vi "automated_scan_v1.0.vi"() -> ()   [LabVIEW 2018]
uses:
  Other_Libraries/MoCo Software/VI/global_m.vi
  <vilib>/Utility/file.llb/Write Delimited Spreadsheet (DBL).vi
  <vilib>/Utility/file.llb/Write Delimited Spreadsheet (string).vi
  Other_Libraries/Thorlabs_FW102C/Thorlabs_FW102C.lvlib
panel:
  out "End scan":errorcluster
  out "nloops":i32
  out "FW Position":i32
  out "Filter Wheel":errorcluster
  out "Current Wavelength(nm)":dbl
  out "Take Image":errorcluster
  out "Dark Integrating Time (s)":dbl caption="Elapsed Time (s)"
  out "% complete":dbl
  out "Total Steps":dbl
  in  "Tab Control":T1(tab)
  in  "Photodiode (VISA resource name)[Com3]":refnum<visa-resource-name>="COM3"
  in  "Mono port":refnum<visa-resource-name>="COM2"
  in  "Grating, gr/mm":u16(ring)=2 items=["2400", "1800", "1200", "600", "300", "150"]
  in  "Take Image":bool=TRUE
  in  "Two Cameras":bool=TRUE
  in  "Step Size":dbl=10.0
  in  "Stop Wavelength":dbl=600.0
  in  "Start Wavelength":dbl=500.0
  in  "Scan Directory":string="Peter_ferguson\\Tcal\\scans\\"
  in  "Scan Name":string="test_scan"
  in  "Scan Type":string(combo)="New Scan"
  in  "Photodiode / Camera\n Integration time(s)":dbl=10.0
  in  "Spectrometer Integration time":dbl=0.001
  out "VISA out":refnum<visa-resource-name>
  out "Current Value Bin":dbl format="%.6f"
  out "dup VISA session":refnum<visa-resource-name>
  out "dup VISA session 2":refnum<visa-resource-name>
  out "Mono wav":dbl format="%.3f"
  out "Photodiode 2":errorcluster
  out "Light Integrating Time (s)":dbl caption="Elapsed Time (s)"
  out "Active Wavelength":u32
  out "Serial Number":string
  out "Mono/Photodiode":errorcluster
  out "Step #":i32
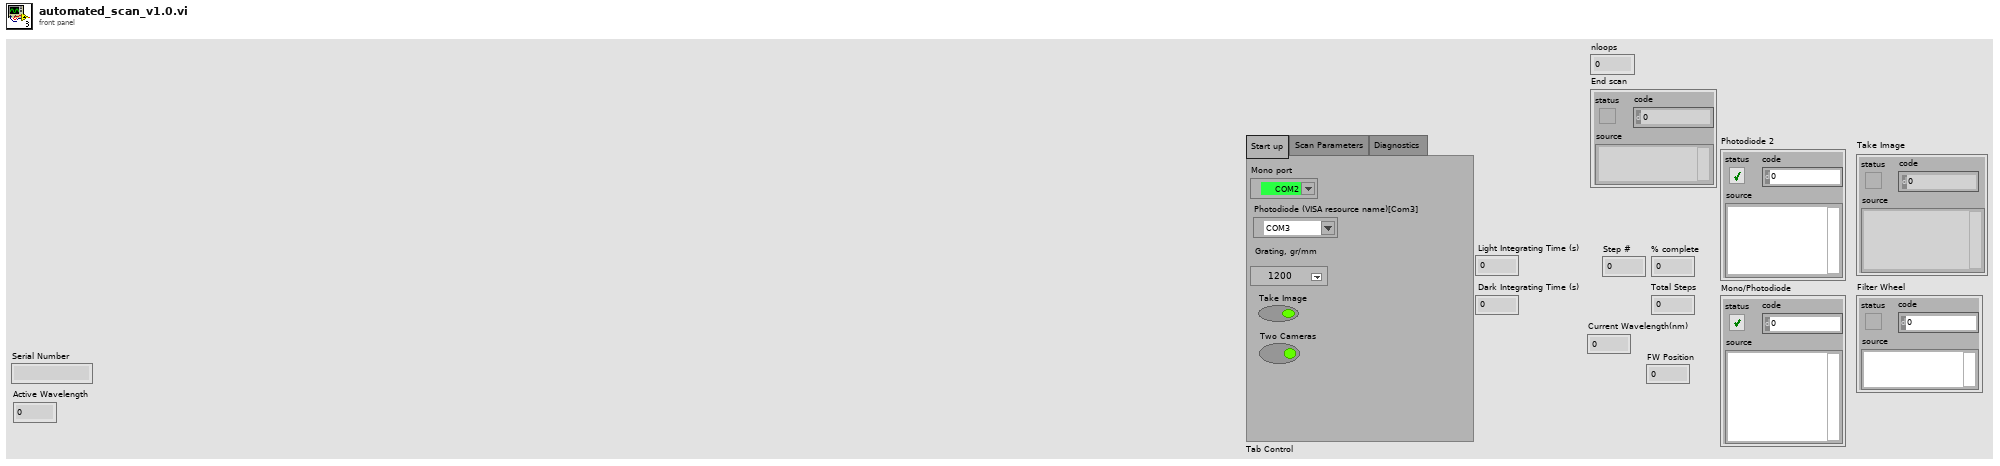
[diagram p1: front panel]
types:
  T1 = enum32{"Start up", "Scan Parameters", "Diagnostics"}
  T2 = cluster{"Head Type":u32, "Head Version":u32, "Serial Number":string, "Calibration Sensitivity":dbl, "Default Wavelength":u32, "Active Sensitivity":dbl, "Active Wavelength":u32, "Scale Min Power (Wattmeter)":u32, "Scale Max Power (Wattmeter)":u32, "Scale Min Energy":u32, "Scale Max Energy":u32, "Current Scale":u32, "Calo Mode":bool, "Anticipation":bool, "External Trig":bool, "Trig Level":dbl, "Zero Offset":dbl, "Multiplier 1":dbl, "Offset 1":dbl, "Multiplier 2":dbl, "Offset 2":dbl, "Max Power (Joulemeter)":dbl, "Max energy (Joulemeter)":dbl, "Currently Logging":bool, "Analog Out Active":bool, "Resolution":dbl, "Currently Calculating Stats":bool, "High-Resolution Display":bool, "Scale Min Wavelenght":u32, "Scale Max Wavelenght":u32, "Upper Bound":dbl, "Lower Bond":dbl, "Reference Value":dbl, "Thresholds Active":bool, "Fail":bool, "Attenuator":bool, "autoScale":bool, "IsdBm":bool}
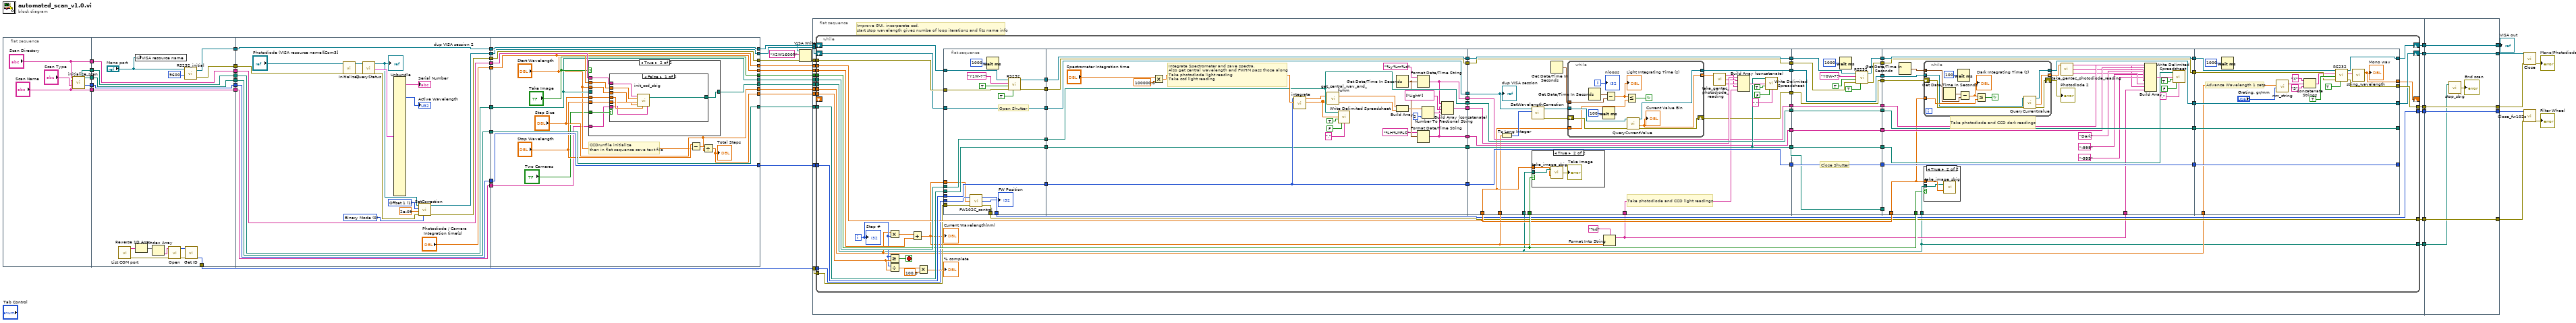
[diagram p0: block diagram]
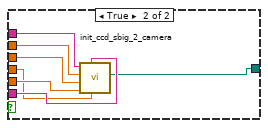
[diagram p5: hidden frame]
diagram:
  n1 = flat-sequence {
    tunnel: [w55] -> w38
    tunnel: [w54] -> w37
    tunnel: [w53] -> w36
    tunnel: ["Scan Directory"] -> w22
    tunnel: ["Scan Name"] -> w7
    tunnel: [w71] -> w35
    tunnel: [w70] -> w34
    tunnel: w38 -> [w69]
    tunnel: [w69] -> w33
    tunnel: w37 -> [w68]
    tunnel: [w68] -> w32
    tunnel: w36 -> [w67]
    tunnel: [w67] -> w31
    tunnel: w22 -> [w66]
    tunnel: [w66] -> w20
    tunnel: [w59] -> w14
    tunnel: [w58] -> w13
    tunnel: [w57] -> w8
    tunnel: w7 -> [w57]
    tunnel: w35 -> [w87]
    tunnel: [w87] -> w30
    tunnel: w34 -> [w83]
    tunnel: w33 -> [w86]
    tunnel: [w86] -> w29
    tunnel: w32 -> [w85]
    tunnel: [w85] -> w28
    tunnel: w31 -> [w84]
    tunnel: [w84] -> w27
    tunnel: [w80] -> w26
    tunnel: ["Photodiode / Camera\n Integration time(s)"] -> w25
    tunnel: [w76] -> w24
    tunnel: [w82] -> w21
    tunnel: w20 -> [w82]
    tunnel: [w74] -> w9
    tunnel: w8 -> [w74]
    tunnel: [w109] -> w40
    tunnel: w30 -> [w109]
    tunnel: [w99] -> w48
    tunnel: w29 -> [w99]
    tunnel: [w108] -> w47
    tunnel: w28 -> [w108]
    tunnel: [w107] -> w46
    tunnel: w27 -> [w107]
    tunnel: [w106] -> w45
    tunnel: w26 -> [w106]
    tunnel: [w103] -> w44
    tunnel: w25 -> [w103]
    tunnel: [w110] -> w39
    tunnel: w24 -> [w105]
    tunnel: [w105] -> w23
    tunnel: w21 -> [w104]
    tunnel: [w101] -> w19
    tunnel: ["Take Image"] -> w18
    tunnel: ["Step Size"] -> w16
    tunnel: ["Start Wavelength"] -> w15
    tunnel: w9 -> [w95]
    frame #0 {
      n2 = call "initialize_scan.vi"("Scan Directory"="Scan Directory", "Scan Name"="Scan Name", "Scan Type"="Scan Type") -> ("Path Spec"=w55:path, "Path Scan"=w53:path, "Wrapper Out"=w54:u64)  [unwired: 8 in, 2 out]
    }
    frame #1 {
      n3 = call "List COM port.vi"() -> ("error out"=w60:errorcluster, "COM Ports"=w63:string[])  [unwired: 10 in]
      n4 = global write "global_m.vi" "VISA resource name"("Mono port") -> ()
      n5 = Reverse 1D Array(array=w63) -> (reversed array=w62:string[])
      n6 = Index Array(array=w62) -> (element=w61:string)  [unwired: 1 in]
      n7 = call "Open.vi"("error in (no error)"=w60, "Serial Port"=w61) -> ("error out"=w64:errorcluster, "FW102C out"=w65:i32)  [unwired: 7 in, 1 out]
      n8 = call "RS232_initial.vi"("baud rate"=u32 9600, "VISA resource name"="Mono port") -> ("error out"=w70:errorcluster, "VISA name out"=w71:refnum<visa-resource-name>)  [unwired: 2 in]
      n9 = call "Get ID.vi"("error in (no error)"=w64, "FW102C in"=w65) -> ("error out"=w58:errorcluster, "FW102C out"=w59:i32)  [unwired: 7 in, 1 out]
    }
    frame #2 {
      w75 = u16 0 items=["Binary Mode", "Text Mode"] ("Transfer Type (binary)")
      w79 = u16 1 items=["Multiplier1", "Offset 1", "Multiplier 2", "Offset 2"] ("Correction Type")
      n10 = call "Initialize2.vi"("error in (no error)"=w83, "Instr. Descriptor (GPIB::)"="Photodiode (VISA resource name)[Com3]") -> ("error out"=w89:errorcluster, "VISA session"=w93:refnum<visa-resource-name>)  [unwired: 4 in]
      n11 = call "QueryStatus.vi"("error in (no error)"=w89, "VISA session"=w93) -> ("error out"=w77:errorcluster, "Status Data"=w92:T2, "dup VISA session"=w81:refnum<visa-resource-name>)  [unwired: 4 in, 1 out]
      "dup VISA session 2" <- w81
      n12 = Unbundle(w92) -> ("Serial Number"=→"Serial Number":string, "Active Wavelength"=→"Active Wavelength":u32)  [unwired: 36 out]
      n13 = call "SetCorrection.vi"("Transfer Type (binary)"=w75, "error in (no error)"=w77, "Correction  Value"=2e-09, "Correction Type"=w79, "VISA session"=w81) -> ("error out"=w76:errorcluster, "dup VISA session"=w80:refnum<visa-resource-name>)  [unwired: 3 in]
    }
    frame #3 {
      # "CCDrunfile initialize\nthen in flat sequence save text file"
      n14 = case shown="True" "Take Image" {
        tunnel: w104 -> [_ w120]
        tunnel: w103 -> [_ w119]
        tunnel: "Step Size" -> [_ w118]
        tunnel: "Stop Wavelength" -> [_ w117]
        tunnel: [w112 w116] -> w101
        tunnel: "Start Wavelength" -> [_ w115]
        tunnel: w99 -> [w112 _]
        tunnel: "Two Cameras" -> [_ w114]
        tunnel: w95 -> [_ w113]
        frame False {
        }
        frame True {
          n15 = case shown="False" w114 {
            tunnel: w120 -> [w127 w134]
            tunnel: w119 -> [w126 w132]
            tunnel: w118 -> [w125 w129]
            tunnel: w117 -> [w124 w130]
            tunnel: [w123 w128] -> w116
            tunnel: w115 -> [w122 w131]
            tunnel: w113 -> [w121 w133]
            frame False {
              n16 = call "init_ccd_sbig.vi"("Scan Directory"=w127, "Exposure Time"=w126, "Min nm"=w122, "Max nm"=w124, "Step size"=w125, "Scan_prefix"=w121) -> ("Working Directory"=w123:path)
            }
            frame True {
              n17 = call "init_ccd_sbig_2_camera.vi"("Step size"=w129, "Scan Prefix"=w133, "Max nm"=w130, "Min nm"=w131, "Exposure Time"=w132, "Scan Directory"=w134) -> ("Working Directory"=w128:path)  [unwired: 3 in]
            }
          }
        }
      }
      n18 = Subtract(x="Stop Wavelength", y="Start Wavelength") -> (x-y=w111:dbl)
      n19 = Divide(x=w111, y="Step Size") -> (x/y=w110:dbl)
      "Total Steps" <- w110
    }
  }
  n20 = VISA Write(VISA resource name=w40, write buffer="X2W1600R", error in (no error)=w23) -> (error out=w49:errorcluster)  [unwired: 2 out]
  n21 = flat-sequence {
    tunnel: w49 -> [w154]
    tunnel: w48 -> [w153]
    tunnel: w47 -> [w152]
    tunnel: w46 -> [w151]
    tunnel: w45 -> [w150]
    tunnel: w44 -> [w149]
    tunnel: w40 -> [w146]
    tunnel: w39 -> [w145]
    tunnel: w19 -> [w144]
    tunnel: w18 -> [w143]
    tunnel: w16 -> [w141]
    tunnel: w15 -> [w140]
    tunnel: w14 -> [w139]
    tunnel: w13 -> [w138]
    tunnel: [w148] -> w6
    tunnel: [w147] -> w5
    tunnel: [w142] -> w4
    tunnel: [w137] -> w3
    tunnel: [w136] -> w2
    tunnel: [w135] -> w1
    tunnel: [w385] -> w10
    tunnel: [w386] -> w11
    tunnel: [w387] -> w17
    tunnel: [w388] -> w41
    tunnel: [w389] -> w43
    tunnel: w6 -> [w389]
    tunnel: w5 -> [w388]
    tunnel: w4 -> [w387]
    tunnel: w3 -> [w386]
    tunnel: w2 -> [w385]
    tunnel: w1 -> [w384]
    frame #0 {
      # "Improve GUI, incorperate ccd,\nstart stop wavelength gives numbe of loop iterations and fits name info"
      n22 = while {
        tunnel: w154 -> [w222]
        tunnel: [w221] -> w148
        tunnel: w153 -> [w220]
        tunnel: w152 -> [w219]
        shift-right: [w173] -> _
        shift-left: _ -> [_]
        tunnel: w151 -> [w206]
        tunnel: w149 -> [w164]
        shift-right: [w174] -> w142
        shift-left: w150 -> [w196]
        shift-right: [w177] -> w147
        shift-left: w146 -> [w175]
        tunnel: w145 -> [w172]
        tunnel: w144 -> [w155]
        tunnel: w143 -> [w168]
        tunnel: w141 -> [w156]
        tunnel: w140 -> [w167]
        tunnel: w139 -> [w162]
        tunnel: w138 -> [w161]
        tunnel: [w159] -> w136
        tunnel: [w158] -> w137
        tunnel: [w155] -> w135
        i -> [w165]
        stop <- w185 stop-if-true
        n23 = Multiply(x=w156, y=w165) -> (x*y=w166:dbl)
        n24 = Greater Or Equal?(x=w165, y=w172) -> (x >= y?=w185:bool)
        n25 = Divide(x=w165, y=w172) -> (x/y=w171:dbl)
        n26 = Add(x=w166, y=w167) -> (x+y=w160:dbl)
        "Current Wavelength(nm)" <- w160
        n27 = Multiply(x=w171, y=100.0) -> (x*y=→"% complete":dbl)
        n28 = flat-sequence {
          tunnel: w222 -> [w239]
          tunnel: [w238] -> w218
          tunnel: [w237] -> w217
          tunnel: [w233] -> w216
          tunnel: w220 -> [w233]
          tunnel: w219 -> [w232]
          tunnel: [w232] -> w215
          tunnel: w206 -> [w231]
          tunnel: [w231] -> w205
          tunnel: w196 -> [w230]
          tunnel: [w230] -> w195
          tunnel: w175 -> [w229]
          tunnel: w162 -> [w228]
          tunnel: w161 -> [w227]
          tunnel: w160 -> [w226]
          tunnel: [w225] -> w159
          tunnel: [w224] -> w158
          tunnel: w218 -> [w266]
          tunnel: [w266] -> w204
          tunnel: w217 -> [w265]
          tunnel: [w265] -> w203
          tunnel: w216 -> [w257]
          tunnel: [w257] -> w202
          tunnel: w215 -> [w258]
          tunnel: [w258] -> w200
          tunnel: w205 -> [w246]
          tunnel: [w246] -> w198
          tunnel: [w245] -> w197
          tunnel: w195 -> [w244]
          tunnel: [w244] -> w194
          tunnel: [w242] -> w184
          tunnel: [w241] -> w179
          tunnel: w204 -> [w292]
          tunnel: w203 -> [w279]
          tunnel: w202 -> [w294]
          tunnel: [w294] -> w201
          tunnel: w200 -> [w293]
          tunnel: [w293] -> w199
          tunnel: w198 -> [w278]
          tunnel: w197 -> [w283]
          tunnel: w194 -> [w291]
          tunnel: [w292] -> w193
          tunnel: w164 -> [w271]
          tunnel: [w279] -> w192
          tunnel: [w278] -> w191
          tunnel: [w277] -> w189
          tunnel: [w276] -> w186
          tunnel: w184 -> [w275]
          tunnel: [w275] -> w183
          tunnel: [w274] -> w180
          tunnel: w179 -> [w274]
          tunnel: w155 -> [w272]
          tunnel: w168 -> [w270]
          tunnel: w157 -> [w267]
          tunnel: w160 -> [w269]
          tunnel: [w323] -> w214
          tunnel: [w322] -> w212
          tunnel: w201 -> [w318]
          tunnel: [w318] -> w210
          tunnel: [w317] -> w208
          tunnel: w199 -> [w317]
          tunnel: w193 -> [w316]
          tunnel: w192 -> [w315]
          tunnel: w191 -> [w310]
          tunnel: [w310] -> w190
          tunnel: w189 -> [w314]
          tunnel: [w314] -> w188
          tunnel: [w313] -> w187
          tunnel: w186 -> [w313]
          tunnel: w183 -> [w312]
          tunnel: [w312] -> w182
          tunnel: [w311] -> w181
          tunnel: w180 -> [w311]
          tunnel: [w310] -> w178
          tunnel: w214 -> [w351]
          tunnel: [w351] -> w213
          tunnel: w212 -> [w350]
          tunnel: [w350] -> w211
          tunnel: w210 -> [w349]
          tunnel: [w349] -> w209
          tunnel: w208 -> [w348]
          tunnel: [w348] -> w207
          tunnel: w190 -> [_]
          tunnel: w188 -> [w333]
          tunnel: w187 -> [w332]
          tunnel: w164 -> [w329]
          tunnel: w182 -> [w340]
          tunnel: w181 -> [w339]
          tunnel: w178 -> [w338]
          tunnel: [w331] -> w176
          tunnel: w155 -> [w328]
          tunnel: w168 -> [w327]
          tunnel: w157 -> [w325]
          tunnel: w213 -> [w379]
          tunnel: w211 -> [w380]
          tunnel: w209 -> [w369]
          tunnel: w207 -> [w371]
          tunnel: [w378] -> w177
          tunnel: [w377] -> w221
          tunnel: [w371] -> _
          tunnel: [w369] -> _
          tunnel: [w368] -> w174
          tunnel: w176 -> [w368]
          tunnel: [w367] -> w173
          tunnel: w156 -> [w366]
          frame #0 {
            # "Open Shutter"
            n29 = call "FW102C_control.vi"("error in (no error)"=w227, "Current Wavelength"=w226, "FW102C in"=w228) -> ("error out"=w224:errorcluster, "Position"=→"FW Position":i32, "FW102C out"=w225:i32)
            n30 = Wait (ms)(milliseconds to wait=u32 1000) -> ()  [unwired: 1 out]
            n31 = call "RS232.vi"("read"=TRUE, "error in"=w239, "write"=TRUE, "string to write"="Y1W-7?" ("string"), "VISA  name in"=w229) -> ("error out"=w237:errorcluster, "VISA out"=w238:refnum<visa-resource-name>)  [unwired: 1 in, 2 out]
          }
          frame #1 {
            # "Integrate Spectrometer and save spectra, \nAlso get central wavelength and FWHM pass those along\nTake photodiode light reading \nTake ccd light reading"
            n32 = Multiply(x="Spectrometer Integration time", y=100000.0) -> (x*y=w262:dbl)
            n33 = call "integrate.vi"("Numeric"=w262, "Wrapper Out"=w258) -> ("Spectrum Values"=w255:dbl[], "WL Values"=w256:dbl[])  [unwired: 7 in, 1 out]
            n34 = call "get_central_wav_and_fwhm.vi"("Signal"=w255, "Wavelenghs"=w256) -> ("FWHM"=w251:dbl, "Central"=w243:dbl)
            n35 = call-poly <vilib>:"Write Delimited Spreadsheet.vi"("file path (dialog if empty)"=w257, "1D data"=w255, "append to file? (new file:F)"=TRUE, "transpose? (no:F)"=FALSE, "delimiter (\\t)"="," ("delimiter (\\t)")) -> ()  [unwired: 9 in, 2 out]
            n36 = Get Date/Time In Seconds() -> (seconds since 1Jan1904=w253:timestamp)
            n37 = Build Array(w243, w251) -> (w250:dbl[])
            n38 = Format Date/Time String(time format string (%c)="%y%m%d", seconds (now)=w253) -> (date/time string=w242:string)  [unwired: 1 in]
            n39 = Format Date/Time String(time format string (%c)="%H%M%S", seconds (now)=w253) -> (date/time string=w241:string)  [unwired: 1 in]
            n40 = Number To Fractional String(number=w250, precision (6)=i16 2) -> (F-format string=w247:string[])  [unwired: 2 in]
            n41 = Build Array (concatenate)(w242, w241, string[] ["Light"] ("array"), w247) -> (w245:string[])
          }
          frame #2 {
            # "Take photodiode and CCD light readings"
            n42 = To Long Integer(number=w269) -> (32bit integer=w290:i32)
            n43 = call "SetWavelengthCorrection.vi"("Wave Length  ( 0= restore default)"=w290, "VISA session"=w291) -> ("error out"=w288:errorcluster, "dup VISA session"=w289:refnum<visa-resource-name>)  [unwired: 6 in]
            n44 = case shown="True" w270 {
              tunnel: w272 -> [_ w297]
              tunnel: w271 -> [_ w296]
              frame False {
              }
              frame True {
                n45 = call "take_image_sbig.vi"("Exptime"=w296, "path"=w297) -> ("error out"=→"Take Image":errorcluster)
              }
            }
            n46 = Get Date/Time In Seconds() -> (seconds since 1Jan1904=w273:timestamp)
            n47 = while {
              tunnel: w289 -> [w309]
              shift-right: [w307] -> w276
              shift-left: w288 -> [w308]
              tunnel: w271 -> [w305]
              tunnel: [w304] -> w284 mode=indexing
              tunnel: [w303] -> w277
              tunnel: w273 -> [w301]
              i -> [w299]
              stop <- w306 continue-if-true
              n48 = Get Date/Time In Seconds() -> (seconds since 1Jan1904=w302:timestamp)
              n49 = Wait (ms)(milliseconds to wait=u32 100) -> ()  [unwired: 1 out]
              n50 = Subtract(x=w302, y=w301) -> (x-y=w300:dbl)
              "Light Integrating Time (s)" <- w300
              n51 = Less Or Equal?(x=w300, y=w305) -> (x <= y?=w306:bool)
              n52 = call "QueryCurrentValue.vi"("error in (no error)"=w308, "VISA session"=w309) -> ("error out"=w307:errorcluster, "Current Value Bin"=w304:dbl, "dup VISA session"=w303:refnum<visa-resource-name>)  [unwired: 3 in, 2 out]
              "Current Value Bin" <- w304
              "nloops" <- w299
            }
            n53 = call "take_gentec_photodiode_reading.vi"("numeric array"=w284) -> ("SD"=w281:string, "Mean"=w282:string, "Num of readings"=w268:string)  [unwired: 2 in]
            n54 = Build Array (concatenate)(w283, w282, w281, w268, w267) -> (w280:string[])
            n55 = call-poly <vilib>:"Write Delimited Spreadsheet.vi"("file path (dialog if empty)"=w278, "1D data"=w280, "append to file? (new file:F)"=TRUE, "transpose? (no:F)"=FALSE, "delimiter (\\t)"="," ("delimiter (\\t)")) -> ()  [unwired: 9 in, 2 out]
            "dup VISA session" <- w291
          }
          frame #3 {
            # "Close Shutter"
            n56 = Wait (ms)(milliseconds to wait=u32 1000) -> ()  [unwired: 1 out]
            n57 = call "RS232.vi"("read"=TRUE, "error in"=w315, "write"=TRUE, "string to write"="Y0W-7?" ("string"), "VISA  name in"=w316) -> ("error out"=w322:errorcluster, "VISA out"=w323:refnum<visa-resource-name>)  [unwired: 1 in, 2 out]
          }
          frame #4 {
            # "Take photodiode and CCD dark readings"
            n58 = Get Date/Time In Seconds() -> (seconds since 1Jan1904=w330:timestamp)
            n59 = while {
              shift-right: [w363] -> w343
              shift-left: w332 -> [w364]
              tunnel: [w361] -> w344 mode=indexing
              tunnel: w329 -> [w360]
              tunnel: w333 -> [w359]
              tunnel: [w358] -> w331
              tunnel: w330 -> [w356]
              stop <- w362 continue-if-true
              n60 = Get Date/Time In Seconds() -> (seconds since 1Jan1904=w357:timestamp)
              n61 = Wait (ms)(milliseconds to wait=u32 100) -> ()  [unwired: 1 out]
              n62 = Subtract(x=w357, y=w356) -> (x-y=w355:dbl)
              "Dark Integrating Time (s)" <- w355
              n63 = Less Or Equal?(x=w355, y=w360) -> (x <= y?=w362:bool)
              n64 = call "QueryCurrentValue.vi"("error in (no error)"=w364, "VISA session"=w359) -> ("error out"=w363:errorcluster, "Current Value Bin"=w361:dbl, "dup VISA session"=w358:refnum<visa-resource-name>)  [unwired: 3 in, 2 out]
            }
            "Photodiode 2" <- w343
            n65 = case shown="True" w327 {
              tunnel: w329 -> [_ w353]
              tunnel: w328 -> [_ w352]
              frame False {
              }
              frame True {
                n66 = call "take_image_sbig.vi"("Exptime"=w353, "path"=w352) -> ()  [unwired: 1 out]
              }
            }
            n67 = call "take_gentec_photodiode_reading.vi"("numeric array"=w344) -> ("SD"=w337:string, "Mean"=w336:string, "Num of readings"=w326:string)  [unwired: 2 in]
            n68 = Build Array(w340, w339, "Dark" ("date/time string"), "-999" ("element"), "-999" ("element"), w336, w337, w326, w325) -> (w341:string[])
            n69 = call-poly <vilib>:"Write Delimited Spreadsheet.vi"("file path (dialog if empty)"=w338, "1D data"=w341, "append to file? (new file:F)"=TRUE, "transpose? (no:F)"=FALSE, "delimiter (\\t)"="," ("delimiter (\\t)")) -> ()  [unwired: 9 in, 2 out]
          }
          frame #5 {
            # "Advance Wavelength 1 setp"
            n70 = Wait (ms)(milliseconds to wait=u32 1000) -> ()  [unwired: 1 out]
            n71 = call "nm_string.vi"("Grating, gr/mm"="Grating, gr/mm", "Wavelength, nm"=w366) -> ("nm_String"=w376:string)  [unwired: 2 in, 1 out]
            n72 = Concatenate Strings("X" ("string"), w376, "S" ("string")) -> (w373:string)
            n73 = call "RS232.vi"("read"=TRUE, "error in"=w380, "write"=TRUE, "string to write"=w373, "VISA  name in"=w379) -> ("error out"=w377:errorcluster, "read string"=w370:string, "VISA out"=w378:refnum<visa-resource-name>)  [unwired: 1 in, 1 out]
            n74 = call "string_wavelength.vi"("Position String"=w370) -> ("Present Wavelength"=w367:dbl)  [unwired: 3 in, 1 out]
            "Mono wav" <- w367
          }
        }
        n75 = Format Into String(format string="%d", w160) -> (resulting string=w157:string)  [unwired: 2 in, 1 out]
        "Step #" <- w165
      }
    }
    frame #1 {
      n76 = call "stop_sbig.vi"("path"=w384) -> ("error out"=→"End scan":errorcluster)  [unwired: 1 in]
    }
  }
  n77 = call "Close.vi"("VISA session"=w17, "error in (no error)"=w43) -> ("error out"=→"Mono/Photodiode":errorcluster)  [unwired: 13 in]
  n78 = call "Close_fw102c.vi"("error in (no error)"=w11, "FW102C in"=w10) -> ("error out"=→"Filter Wheel":errorcluster)  [unwired: 9 in]
  "VISA out" <- w41
